vi "Module Init.vi"(8 "error in (no error)":errorcluster, 11 "Data Logger BOOL Module in":refnum<class "Data Logger BOOL Module.lvclass">) -> (0 "error out":errorcluster, 3 "Data Logger BOOL Module out":refnum<class "Data Logger BOOL Module.lvclass">)   [LabVIEW 2020, in "VolatusData.lvlib" / "Data Logger BOOL Module.lvclass"]
uses:
  Data Logger BOOL Module.lvclass
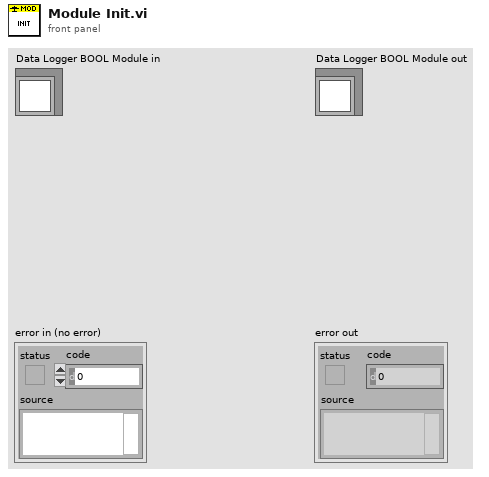
[diagram p1: front panel]
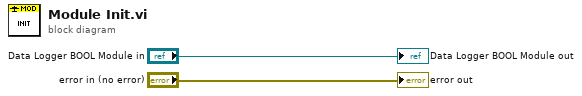
[diagram p0: block diagram]
diagram:
  "error out" <- "error in (no error)"
  "Data Logger BOOL Module out" <- "Data Logger BOOL Module in"
